vi "Teleope Balance 2.vi"   [LabVIEW 2020]
uses:
  <vilib>/Rock Robotics/WPI/Utilities/WPI_GetSetVariantRefNum.vi
  Robot Global Data.vi
  <vilib>/Rock Robotics/WPI/RobotDrive/WPI_RobotDriveArcadeDrive_Standard(NoSaturation).vi
types:
  T1 = typedef "WPI_RobotDriveDevRef.ctl" = cluster{"DevStatus":errorcluster, "Motors[]":T2[], "Square Inputs":bool, "Max Output":dbl}
  T2 = typedef "WPI_MotorControlDeviceRef.ctl" = cluster{"DeviceStatus":errorcluster, "Type":T3, "PWM":cluster{"PWM Channel":T4, "DeadBand":T5}, "CAN":cluster{"Device Number":u8, "SetOutput VI Ref":variant, "GetOutput VI Ref":variant, "Enable VI Ref":variant, "Disable VI Ref":variant, "Data":variant}, "Invert":bool, "DIO PWM":cluster{"PWM \"Enable\" Channel":T4, "DIOChannel":T6, "PWM Rate":dbl}}
  T3 = typedef "WPI_MotorControlType.ctl" = enum16{"PWM", "CAN", "DIO PWM"}
  T4 = typedef "FPGA_DIOPWMChannel.ctl" = enum8{"PWM 0", "PWM 1", "PWM 2", "PWM 3", "PWM 4", "PWM 5", "PWM 6", "PWM 7", "PWM 8", "PWM 9", "PWM MXP 0", "PWM MXP 1", "PWM MXP 2", "PWM MXP 3", "PWM MXP 4", "PWM MXP 5", "PWM MXP 6", "PWM MXP 7", "PWM MXP 8", "PWM MXP 9", "Invalid"}
  T5 = typedef "WPI_PWMDeadband.ctl" = cluster{"Name":string, "maxPositivePwm":i32, "minPositivePwm":i32, "centerPwm":i32, "maxNegativePwm":i32, "minNegativePwm":i32, "angularRange":u16}
  T6 = typedef "FPGA_DIOChannel.ctl" = enum8{"DIO 0", "DIO 1", "DIO 2", "DIO 3", "DIO 4", "DIO 5", "DIO 6", "DIO 7", "DIO 8", "DIO 9", "DIO MXP 0", "DIO MXP 1", "DIO MXP 2", "DIO MXP 3", "DIO MXP 4", "DIO MXP 5", "DIO MXP 6", "DIO MXP 7", "DIO MXP 8", "DIO MXP 9", "DIO MXP 10", "DIO MXP 11", "DIO MXP 12", "DIO MXP 13", "DIO MXP 14", "DIO MXP 15", "SPI Port CS1", "SPI Port CS2", "SPI Port CS3", "SPI Port MISO", "SPI Port MOSI", "Invalid"}
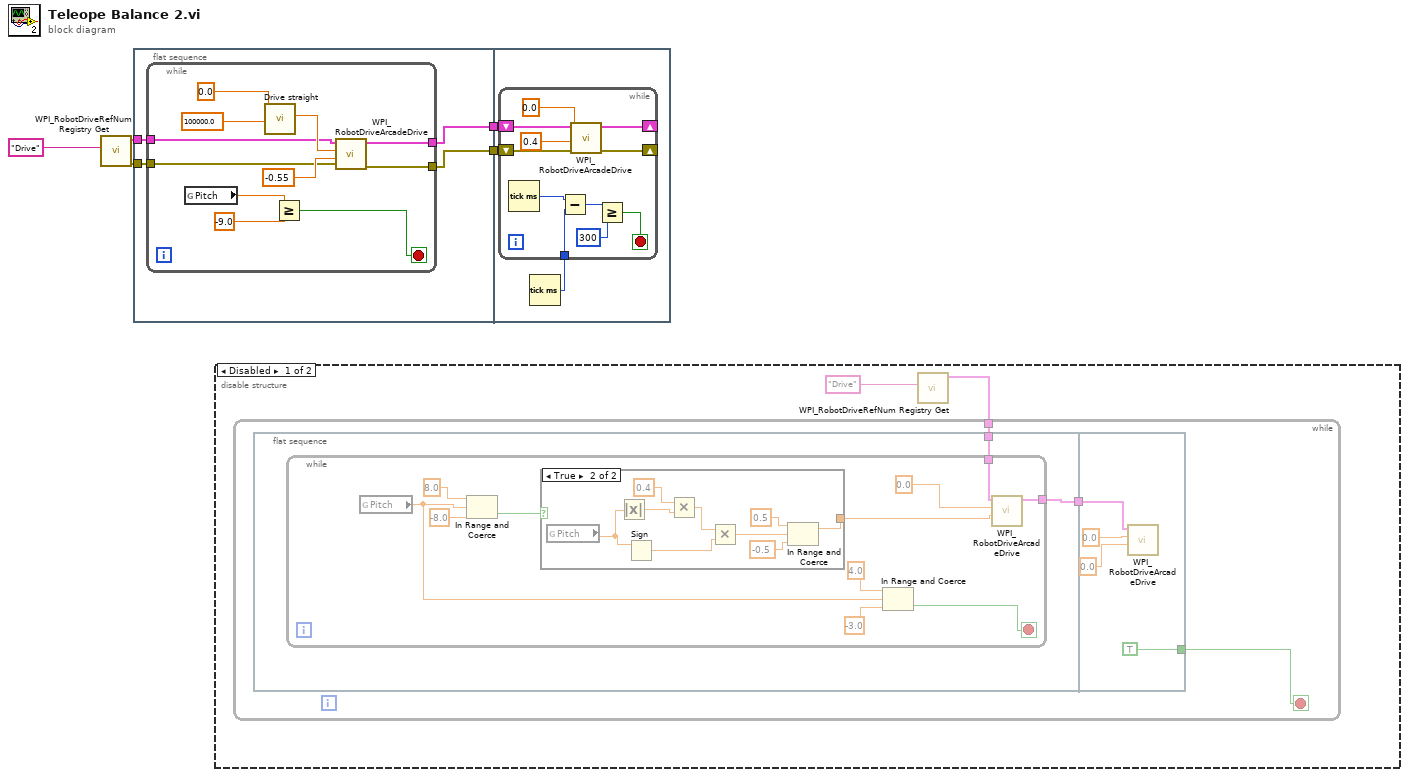
[diagram p0: block diagram]
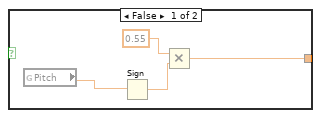
[diagram p2: hidden frame]
diagram:
  n1 = call <vilib>:"WPI_RobotDriveRefNum Registry Get.vi"("refnum name"="Drive") -> ("error out"=w3:errorcluster, "RobotDriveDevRef"=w4:T1)  [unwired: 9 in]
  n2 = flat-sequence {
    tunnel: w4 -> [w9]
    tunnel: w3 -> [w8]
    tunnel: [w7] -> w2
    tunnel: [w6] -> w1
    tunnel: w2 -> [w23]
    tunnel: w1 -> [w22]
    frame #0 {
      n3 = while {
        tunnel: w9 -> [w13]
        tunnel: w8 -> [w12]
        tunnel: [w11] -> w7
        tunnel: [w10] -> w6
        stop <- w14 stop-if-true
        n4 = global read "Robot Global Data.vi" "Pitch"() -> (w18:dbl)
        n5 = call "Drive straight.vi"("Length(seconds)"=100000.0, "Desired angle"=0.0) -> ("X Power"=w16:dbl)  [unwired: 8 in, 1 out]
        n6 = Greater Or Equal?(x=w18, y=-9.0) -> (x >= y?=w14:bool)
        n7 = call-poly <vilib>:"WPI_RobotDriveArcadeDrive.vi"("error in (no error)"=w12, "Y axis value"=-0.55, "X axis value"=w16, "RobotDriveDevRef"=w13) -> ("error out"=w10:errorcluster, "RobotDriveDevRef"=w11:T1)  [unwired: 5 in, 1 out]
      }
    }
    frame #1 {
      n8 = Tick Count (ms)() -> (millisecond timer value=w21:u32)
      n9 = while {
        shift-right: [w32] -> _
        shift-left: w23 -> [w34]
        shift-right: [w31] -> _
        shift-left: w22 -> [w33]
        tunnel: w21 -> [w27]
        stop <- w24 stop-if-true
        n10 = Tick Count (ms)() -> (millisecond timer value=w28:u32)
        n11 = Subtract(x=w28, y=w27) -> (x-y=w26:u32)
        n12 = call-poly <vilib>:"WPI_RobotDriveArcadeDrive.vi"("error in (no error)"=w33, "Y axis value"=0.4, "X axis value"=0.0, "RobotDriveDevRef"=w34) -> ("error out"=w31:errorcluster, "RobotDriveDevRef"=w32:T1)  [unwired: 5 in, 1 out]
        n13 = Greater Or Equal?(x=w26, y=u32 300) -> (x >= y?=w24:bool)
      }
    }
  }
  n14 = disable-structure shown="Disabled" {
    frame Disabled {
      n15 = call <vilib>:"WPI_RobotDriveRefNum Registry Get.vi"("refnum name"="Drive") -> ("RobotDriveDevRef"=w35:T1)  [unwired: 9 in, 1 out]
      n16 = while {
        tunnel: w35 -> [w37]
        stop <- w38 stop-if-true
        n17 = flat-sequence {
          tunnel: [w41] -> w39
          tunnel: w37 -> [w40]
          tunnel: w39 -> [w67]
          tunnel: [TRUE] -> w38
          frame #0 {
            n18 = while {
              tunnel: [w48] -> w41
              tunnel: w40 -> [w47]
              stop <- w49 stop-if-true
              n19 = global read "Robot Global Data.vi" "Pitch"() -> (w42:dbl)
              n20 = In Range and Coerce(upper limit=8.0, x=w42, lower limit=-8.0) -> (In Range?=w44:bool)  [unwired: 1 out]
              n21 = case shown="True" w44 {
                tunnel: [w53 w62] -> w43
                frame False {
                  n22 = global read "Robot Global Data.vi" "Pitch"() -> (w55:dbl)
                  n23 = Sign(1:w55) -> (0:w54:dbl)
                  n24 = Multiply(x=0.55, y=w54) -> (x*y=w53:dbl)
                }
                frame True {
                  n25 = global read "Robot Global Data.vi" "Pitch"() -> (w57:dbl)
                  n26 = Absolute Value(x=w57) -> (abs(x)=w58:dbl)
                  n27 = Sign(1:w57) -> (0:w59:dbl)
                  n28 = Multiply(x=0.4, y=w58) -> (x*y=w61:dbl)
                  n29 = Multiply(x=w61, y=w59) -> (x*y=w60:dbl)
                  n30 = In Range and Coerce(upper limit=0.5, x=w60, lower limit=-0.5) -> (coerced(x)=w62:dbl)  [unwired: 1 out]
                }
              }
              n31 = In Range and Coerce(upper limit=4.0, x=w42, lower limit=-3.0) -> (In Range?=w49:bool)  [unwired: 1 out]
              n32 = call-poly <vilib>:"WPI_RobotDriveArcadeDrive.vi"("Y axis value"=w43, "X axis value"=0.0, "RobotDriveDevRef"=w47) -> ("RobotDriveDevRef"=w48:T1)  [unwired: 6 in, 2 out]
            }
          }
          frame #1 {
            n33 = call-poly <vilib>:"WPI_RobotDriveArcadeDrive.vi"("Y axis value"=0.0, "X axis value"=0.0, "RobotDriveDevRef"=w67) -> ()  [unwired: 6 in, 3 out]
          }
        }
      }
    }
    frame Enabled {
    }
  }
